vi "CARICA PROFILO.vi"(8 "error in (no error)":errorcluster, 10 "Text.Text":string, 11 "Refnum in":T1) -> (0 "error out":errorcluster, 1 "Array":string[](array[string]), 2 "Step profilo":string[][](array[string]), 3 "Refnum out":T1, 4 "tipo_profilo":string, 5 "tipo collegamento":string)   [LabVIEW 2019]
uses:
  <vilib>/addons/database/Connection.llb/Conn ObjectReference.ctl
  <vilib>/addons/database/NI_Database_API.lvlib
panel:
  out "data":string[][](array[string])
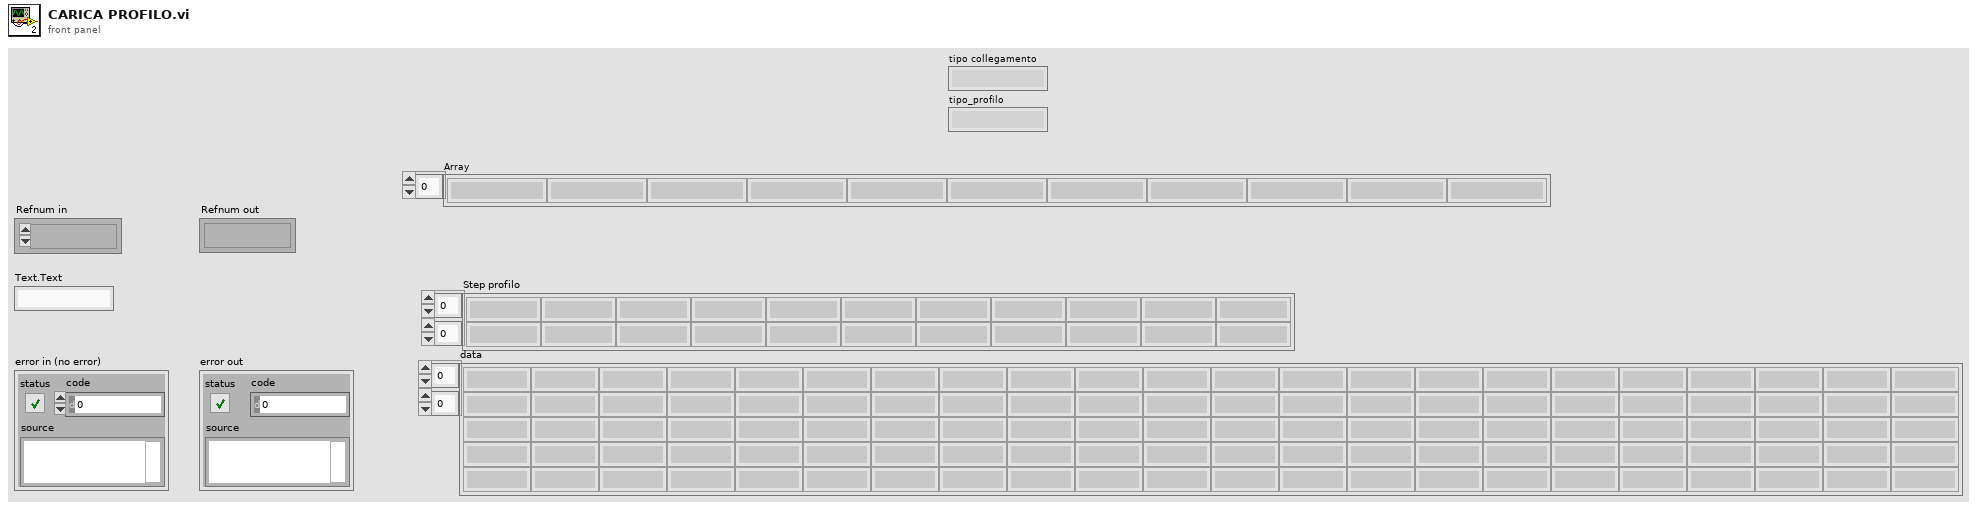
[diagram p1: front panel]
types:
  T1 = typedef "NI_Database_API.lvlib/Conn ObjectReference.ctl" = refnum<k1>
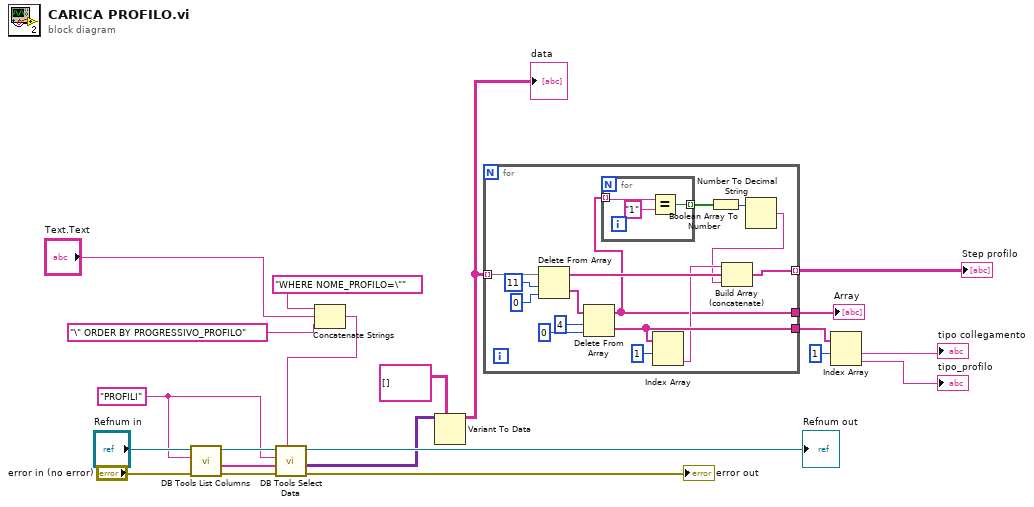
[diagram p0: block diagram]
diagram:
  w9 = "PROFILI" ("table")
  n1 = call <vilib>:"DB Tools List Columns.vi"("error in (no error)"="error in (no error)", "table"=w9, "connection reference"="Refnum in") -> ("error out"=w10:errorcluster, "columns"=w8:string[], "connection reference out"=w12:T1)  [unwired: 1 in, 1 out]
  n2 = Concatenate Strings("WHERE NOME_PROFILO=\"" ("condition"), "Text.Text", "\" ORDER BY PROGRESSIVO_PROFILO" ("string")) -> (w17:string)
  n3 = call <vilib>:"DB Tools Select Data.vi"("condition"=w17, "error in (no error)"=w10, "columns"=w8, "table"=w9, "connection reference"=w12) -> ("error out"=→"error out":errorcluster, "data"=w14:variant[][], "connection reference out"=→"Refnum out":T1)  [unwired: 1 in]
  n4 = Variant To Data(type=string[][] [], Variant=w14) -> (data=w7:string[][])  [unwired: 1 in, 1 out]
  "data" <- w7
  n5 = for {
    tunnel: w7 -> [w36] mode=indexing
    tunnel: [w29] -> w6 mode=indexing
    tunnel: [w25] -> w5
    tunnel: [w27] -> w4
    n6 = Delete From Array(array=w36, length=11, index=0) -> (deleted portion=w33:string[], array with subset deleted=w32:string[])
    n7 = Delete From Array(array=w33, length=4, index=0) -> (deleted portion=w27:string[], array with subset deleted=w25:string[])
    n8 = for {
      tunnel: w25 -> [w39] mode=indexing
      tunnel: [w37] -> w24 mode=indexing
      n9 = Equal?(x=w39, y="1") -> (x = y?=w37:bool)
    }
    n10 = Index Array(array=w27, index #1=1 ("index")) -> (element #2=w26:string)  [unwired: 1 in, 1 out]
    n11 = Boolean Array To Number(Boolean array=w24) -> (number=w23:u32)
    n12 = Number To Decimal String(number=w23) -> (decimal integer string=w22:string)  [unwired: 1 in]
    n13 = Build Array (concatenate)(w26, w32, w22) -> (w29:string[])
  }
  "Step profilo" <- w6
  "Array" <- w5
  n14 = Index Array(array=w4, index #1=1 ("index")) -> (element #1=→"tipo collegamento":string, element #2=→"tipo_profilo":string)  [unwired: 1 in]
